vi "findMostRecentFile.vi"(8 "error in":errorcluster, 11 "Folder Path In":path) -> (0 "error out":errorcluster, 3 "File Path Out":path)   [LabVIEW 2017]
panel:
  # "Overview: This VI takes in a listing of files from a folder path, finds out all the files in the folder, and returns the path to the most recent file.\nRequirements: LabVIEW Base Development System\nInstructions:\n1. Select folder for searching most recent file.\n2. Run VI.\n3. Observe most recent file at File Path Out indicator."
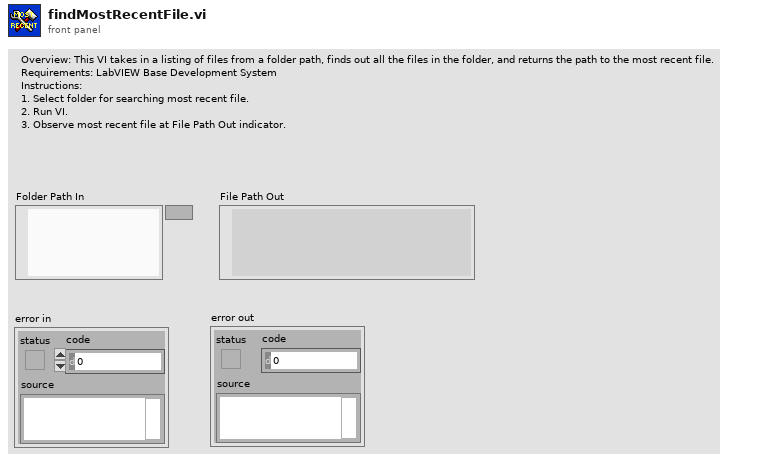
[diagram p1: front panel]
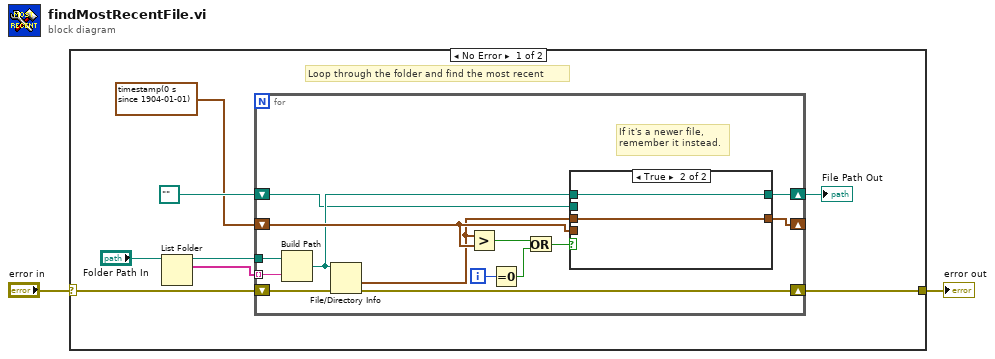
[diagram p0: block diagram]
diagram:
  n1 = case shown="No Error" "error in" {
    selector: "error in" -> [w6 w29]
    tunnel: [w10 w29] -> w2
    frame No Error {
      # "Loop through the folder and find the most recent"
      n2 = List Folder(path="Folder Path In") -> (path out=w3:path, filenames=w4:string[])  [unwired: 3 in, 2 out]
      n3 = for {
        shift-right: [w18] -> _
        shift-left: timestamp(0 s since 1904-01-01) ("last mod 2") -> [w19]
        shift-right: [w15] -> w9
        shift-left: path "" -> [w14]
        shift-right: [w13] -> w10
        shift-left: w6 -> [w24]
        tunnel: w4 -> [w12] mode=indexing
        tunnel: w3 -> [w11]
        i -> [w20]
        # "If it's a newer file,\nremember it instead."
        n4 = Build Path(base path=w11, name or relative path=w12) -> (appended path=w16:path)
        n5 = File/Directory Info(path=w16, error in=w24) -> (last mod=w17:timestamp, error out=w13:errorcluster)  [unwired: 5 out]
        n6 = Greater?(x=w17, y=w19) -> (0:w22:bool)
        n7 = Equal To 0?(x=w20) -> (x = 0?=w21:bool)
        n8 = Or(x=w22, y=w21) -> (x .or. y?=w23:bool)
        n9 = case shown="True" w23 {
          tunnel: w19 -> [w26 _]
          tunnel: [w26 w28] -> w18
          tunnel: w17 -> [_ w28]
          tunnel: w16 -> [_ w27]
          tunnel: [w25 w27] -> w15
          tunnel: w14 -> [w25 _]
          frame False {
          }
          frame True {
          }
        }
      }
      "File Path Out" <- w9
    }
    frame Error {
      # "If there is any error, do not do anything."
    }
  }
  "error out" <- w2
